vi "init camera controller.vi"(6 "Interlock Q Class out":refnum<class "Interlock Q Class.lvclass">, 8 "error in (no error)":errorcluster, 9 "Process State Data out":refnum<data-value>, 10 "Camera Data":refnum<data-value>, 11 "Camera Controller in":refnum<class "Camera Controller.lvclass">) -> (0 "error out":errorcluster, 3 "Camera Controller out":refnum<class "Camera Controller.lvclass">)   [LabVIEW 2022 SP3, in "Camera Controller.lvclass"]
uses:
  Camera Controller.lvclass
  XY Stage/Process Actor/Process Framework/Interlock Q Class/Interlock Q Class.lvclass
  XY Stage/Process Actor/Process Framework/Process State Data/Process State Data.lvclass
  Camera Data/Camera Data.lvclass
  Camera Controller.lvclass/Camera Controller.ctl
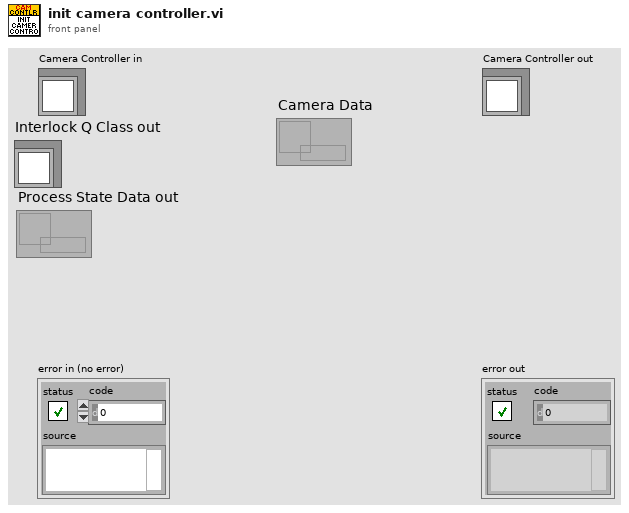
[diagram p1: front panel]
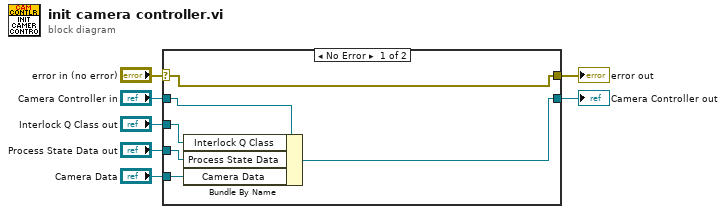
[diagram p0: block diagram]
diagram:
  n1 = case shown="No Error" "error in (no error)" {
    selector: "error in (no error)" -> [w12 w15]
    tunnel: [w12 w15] -> w6
    tunnel: [w11 w14] -> w4
    tunnel: "Camera Controller in" -> [w13 w14]
    tunnel: "Interlock Q Class out" -> [w10 _]
    tunnel: "Process State Data out" -> [w9 _]
    tunnel: "Camera Data" -> [w8 _]
    frame No Error {
      n2 = Bundle By Name(cluster=w13, "Interlock Q Class"=w10, "Process State Data"=w9, "Camera Data"=w8) -> (w11:refnum<class "Camera Controller.lvclass">)
    }
    frame Error {
    }
  }
  "error out" <- w6
  "Camera Controller out" <- w4
